vi "SGTemplate.vi"() -> ()   [LabVIEW 2013]
uses:
  <vilib>/Platform/TimedLoop/XDataNode/timing_clust.ctl
  <vilib>/Platform/TimedLoop/XDataNode/nitl_modes.ctl
  <vilib>/Platform/TimedLoop/XDataNode/wakeup.ctl
  <vilib>/rvi/Emulation/niFpgaSctlEmulationGetInTimedLoop.vi
  <vilib>/rvi/Emulation/niFpgaEmulationReportErrorSimple.vi
  <vilib>/rvi/Emulation/niFpgaGetClockAttributes.vi
  <vilib>/rvi/Emulation/niFpgaCriticalErrorInLSC.vi
  <vilib>/Platform/TimedLoop/XDataNode/XDataNode.xnode
  <vilib>/Platform/TimedLoop/XDataNode/XDNodeRunTimeDep.lvlib
panel:
  in  "SGAmp0":u16
  in  "SGFreq0":u32=100000
  in  "SGPhase0":u32
  in  "AO0":i16
  in  "SGSignalType0":u8
  in  "SGUpdateRate0":u32=40
  in  "AOEnable0":bool
  out "auxAI0":i16
  # "Controls required for\na signal generator"
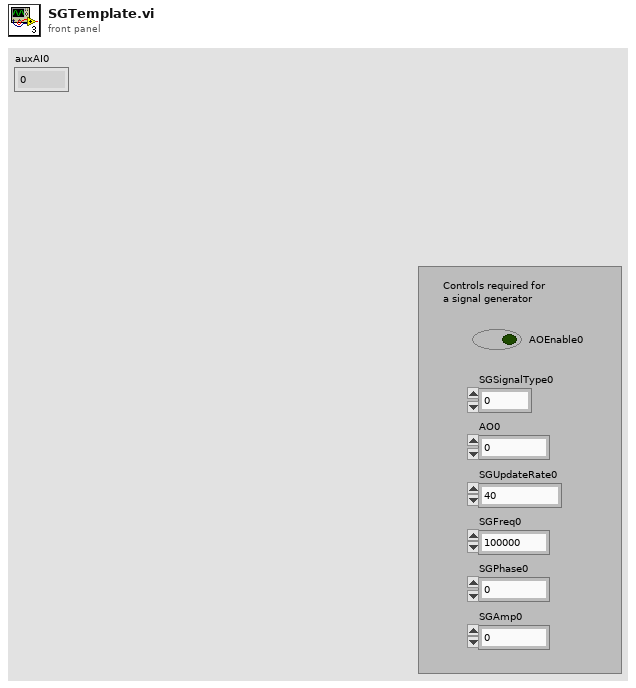
[diagram p1: front panel]
types:
  T1 = typedef "XDNodeRunTimeDep.lvlib/timing_clust.ctl" = cluster{"Expected End [f-1]":u64, "Actual End [f-1]":u64, "Finished Late? [f-1]":bool, "Expected End [i-1]":u64, "Actual End [i-1]":u64, "Finished Late? [i-1]":bool, "Expected Start [i]":u64, "Actual Start [i]":u64, "Expected Start [f]":u64, "Actual Start [f]":u64, "Source Name":string, "Structure Name":string, "Period":i64, "Deadline":i64, "Offset":i64, "Start":i64, "Priority":i32, "Timeout":i32, "Mode":T2, "Wakeup Reason":T3, "Error":errorcluster, "Source Type":string, "Secondary Source Type":string, "Global End Time":u64, "Global Start Time":u64, "Frame Duration":u64, "Iteration Duration":u64, "Assigned CPU":i32, "I/O Scan Engine Mode":u32}
  T2 = typedef "XDNodeRunTimeDep.lvlib/nitl_modes.ctl" = enum32{"No Change", "Process missed periods, maintain original phase", "Discard missed periods, maintain original phase", "Process missed periods, ignore original phase", "Discard missed periods, ignore original phase"}
  T3 = typedef "XDNodeRunTimeDep.lvlib/wakeup.ctl" = enum32{"Normal", "Aborted", "Asynchronous wakeup", "Timing source error", "Timed loop error", "Timeout"}
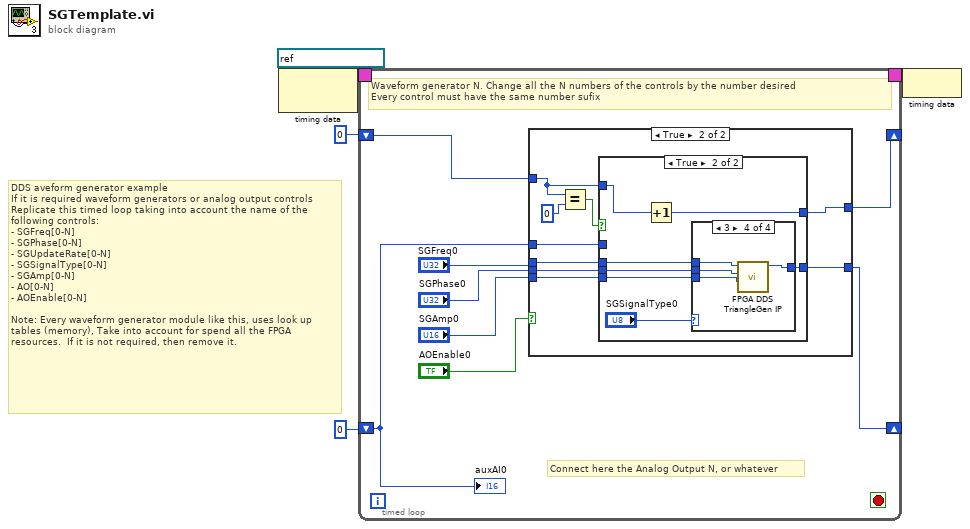
[diagram p0: block diagram]
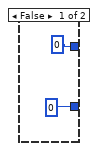
[diagram p2: hidden frame]
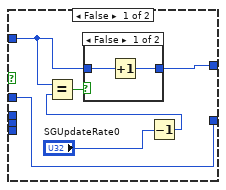
[diagram p3: hidden frame]
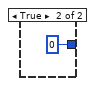
[diagram p4: hidden frame]
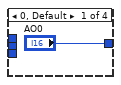
[diagram p5: hidden frame]
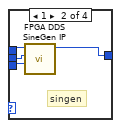
[diagram p6: hidden frame]
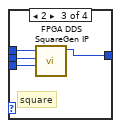
[diagram p7: hidden frame]
diagram:
  # "DDS aveform generator example\nIf it is required waveform generators or analog output controls\nReplicate this timed loop taking into account the name of the \nfollowing controls:\n- SGFreq[0-N]\n- SGPhase[0-N]\n- SGUpdateRate[0-N]\n- SGSignalType[0-N]\n- SGAmp[0-N]\n- AO[0-N]\n- AOEnable[0-N]\n\nNote: Every waveform generator module like this, uses look up tables (memory), Take into account for spend all the FPGA resources.  If it is not required, then remove it."
  n1 = node-c288(refnum<k21> "100 MHz Clock" ("Source Name")) -> (w5:T1)
  n2 = timed-loop {
    shift-right: [w9] -> _
    shift-left: i16 0 ("Signal Value") -> [w6]
    timing: w5 -> [_]
    timing-out: [_] -> w4
    shift-right: [w7] -> _
    shift-left: u32 0 -> [w8]
    stop <- _ stop-if-true
    # "Connect here the Analog Output N, or whatever"
    # "Waveform generator N. Change all the N numbers of the controls by the number desired\nEvery control must have the same number sufix"
    n3 = case shown="True" "AOEnable0" {
      tunnel: "SGFreq0" -> [_ w24]
      tunnel: "SGPhase0" -> [_ w23]
      tunnel: "SGAmp0" -> [_ w22]
      tunnel: [i16 0 w21] -> w9
      tunnel: w8 -> [_ w18]
      tunnel: [u32 0 w17] -> w7
      tunnel: w6 -> [_ w16]
      frame False {
      }
      frame True {
        n4 = Equal?(x=w18, y=u32 0) -> (x = y?=w20:bool)
        n5 = case shown="True" w20 {
          tunnel: w24 -> [_ w40]
          tunnel: w23 -> [_ w39]
          tunnel: w22 -> [_ w38]
          tunnel: [w29 w37] -> w21
          tunnel: w18 -> [w28 w35]
          tunnel: [w30 w34] -> w17
          tunnel: w16 -> [w29 _]
          frame False {
            n6 = Decrement(x="SGUpdateRate0") -> (x-1=w26:u32)
            n7 = Equal?(x=w28, y=w26) -> (x = y?=w27:bool)
            n8 = case shown="False" w27 {
              tunnel: w28 -> [w32 _]
              tunnel: [w31 u32 0] -> w30
              frame False {
                n9 = Increment(x=w32) -> (x+1=w31:u32)
              }
              frame True {
              }
            }
          }
          frame True {
            n10 = Increment(x=w35) -> (x+1=w34:u32)
            n11 = case shown="3" "SGSignalType0" {
              tunnel: w40 -> [_ w45 w49 w53]
              tunnel: w39 -> [_ w44 w48 w52]
              tunnel: w38 -> [_ w43 w47 w51]
              tunnel: ["AO0" w42 w46 w50] -> w37
              frame 0, Default {
              }
              frame 1 {
                # "singen"
                n12 = call "FPGA DDS SineGen IP.vi"("Signal Amplitude (x 2^15)"=w43, "Phase Shift"=w44, "Accumulator Increment"=w45) -> ("Signal Value"=w42:i16)  [unwired: 7 in, 1 out]
              }
              frame 2 {
                # "square"
                n13 = call "FPGA DDS SquareGen IP.vi"("Signal Amplitude (x 2^15)"=w47, "Phase Shift"=w48, "Accumulator Increment"=w49) -> ("Signal Value"=w46:i16)  [unwired: 7 in, 1 out]
              }
              frame 3 {
                n14 = call "FPGA DDS TriangleGen IP.vi"("Signal Amplitude (x 2^15)"=w51, "Phase Shift"=w52, "Accumulator Increment"=w53) -> ("Signal Value"=w50:i16)  [unwired: 7 in, 1 out]
              }
            }
          }
        }
      }
    }
    "auxAI0" <- w6
  }
  n15 = node-c288(w4) -> ()
